vi "Setpoint.vi"(8 "error in (no error)":errorcluster, 10 "Setpoint [A]":dbl format="%.5f", 11 "PS Driver.lvlib:PS Driver.lvclass in":refnum<class "PS Driver.lvclass">) -> (0 "error out":errorcluster, 2 "Setpoint out (A)":dbl, 3 "PS Driver.lvlib:PS Driver.lvclass out":refnum<class "PS Driver.lvclass">)   [LabVIEW 2025, in "PS Driver.lvlib" / "PS Driver.lvclass"]
doc: "Author: Scott Hannahs <sth@magnet.fsu.edu>\n\nThis software is licensed for use under the “MIT License\"\nCopyright (c) 2025 Scott Hannahs, sth@sth@magnet.sthnet.net\n\nPermission is hereby granted, free of charge, to any person obtaining a copy of this software and associated documentation files (the \"Software\"), to deal in the Software without restriction, including without limitation the rights to use, copy, modify, merge, publish, distribute, sublicense, and/or sell copies of the Software, and to permit persons to whom the Software is furnished to do so, subject to the following conditions: The above copyright notice and this permission notice shall be included in all copies or substantial portions of the Software.\n\nTHE SOFTWARE IS PROVIDED \"AS IS\", WITHOUT WARRANTY OF ANY KIND, EXPRESS OR IMPLIED, INCLUDING BUT NOT LIMITED TO THE WARRANTIES OF MERCHANTABILITY, FITNESS FOR A PARTICULAR PURPOSE AND NONINFRINGEMENT. IN NO EVENT SHALL THE AUTHORS OR COPYRIGHT HOLDERS BE LIABLE FOR ANY CLAIM, DAMAGES OR OTHER LIABILITY, WHETHER IN AN ACTION OF CONTRACT, TORT OR OTHERWISE, ARISING FROM, OUT OF OR IN CONNECTION WITH THE SOFTWARE OR THE USE OR OTHER DEALINGS IN THE SOFTWARE."
uses:
  PS Driver.lvclass
  PS Driver.lvclass/PS Driver.ctl
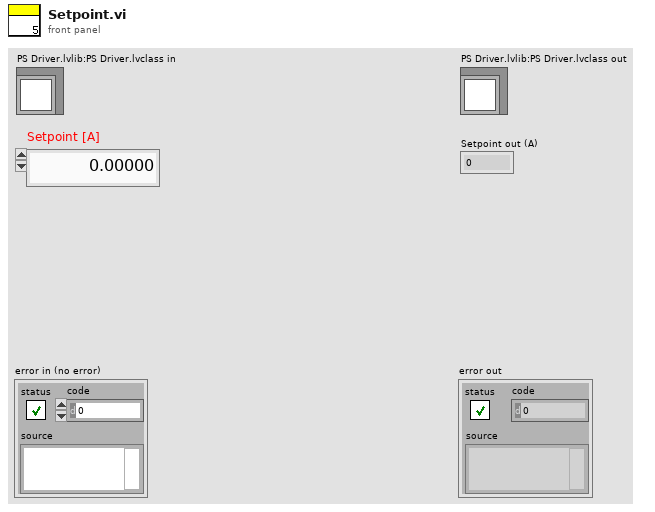
[diagram p1: front panel]
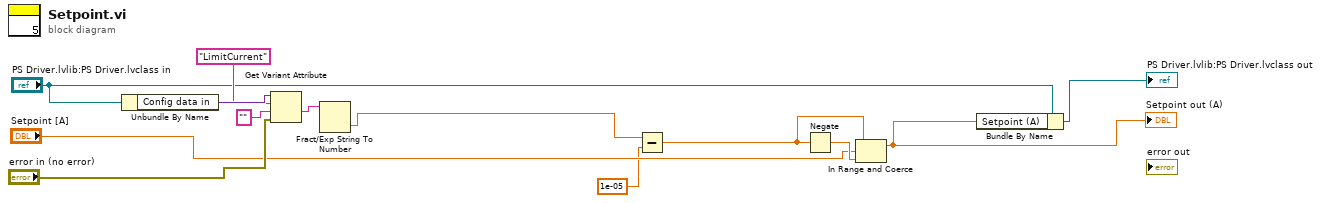
[diagram p0: block diagram]
diagram:
  n1 = Unbundle By Name("PS Driver.lvlib:PS Driver.lvclass in") -> ("Config data in"=w13:variant)
  n2 = Get Variant Attribute(Variant=w13, name="LimitCurrent", default value (empty Variant)="", error in="error in (no error)") -> (value=w9:string)  [unwired: 3 out]
  n3 = Fract/Exp String To Number(string=w9) -> (number=w1:dbl)  [unwired: 3 in, 1 out]
  n4 = Subtract(x=w1, y=1e-05) -> (x-y=w5:dbl)
  n5 = Negate(x=w5) -> (-x=w8:dbl)
  n6 = In Range and Coerce(upper limit=w5, x="Setpoint [A]", lower limit=w8) -> (coerced(x)=w2:dbl)  [unwired: 1 out]
  "Setpoint out (A)" <- w2
  n7 = Bundle By Name(cluster="PS Driver.lvlib:PS Driver.lvclass in", "Setpoint (A)"=w2) -> (→"PS Driver.lvlib:PS Driver.lvclass out":refnum<class "PS Driver.lvclass">)
